vi "Msg.vi"(7 "Actor in":refnum<class "Actor.lvclass">, 11 "Actor Create Msg Strategy in":refnum<class "Actor Create Msg Strategy.lvclass">) -> (0 "error out":errorcluster, 5 "Actor out":refnum<class "Actor.lvclass">)   [LabVIEW 2021, in "Actor Create.lvlib" / "Actor Create Msg Strategy.lvclass"]
uses:
  Actor Create Msg Strategy.lvclass
  LVCAM/Actor/Actor.lvclass
  Actor Create/Actor Create.lvclass
  Actor Create Msg Strategy.lvclass/Actor Create Msg Strategy.ctl
  f99a6dc6-f889-48dc-862a-3d2cf2a0d6f5.vi
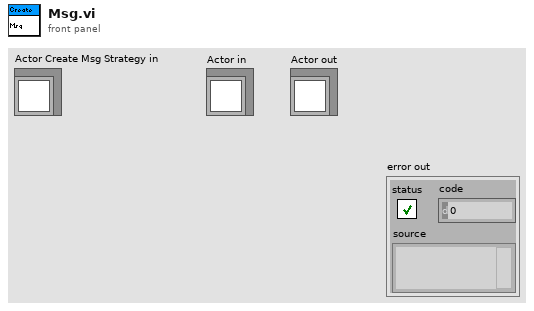
[diagram p1: front panel]
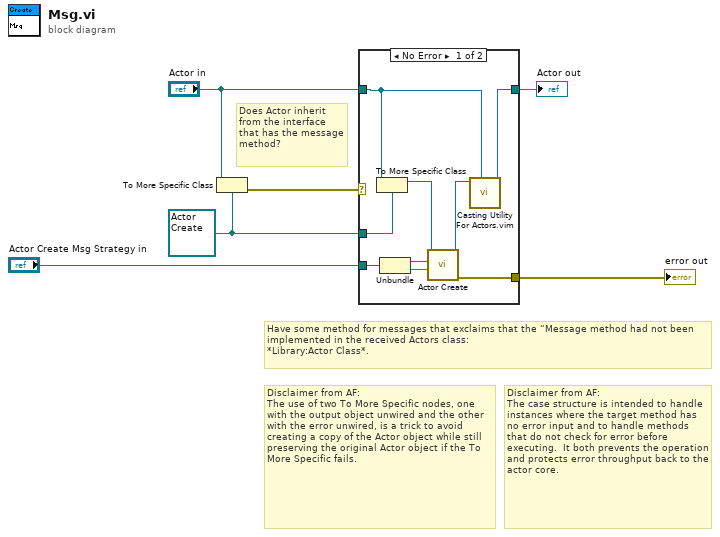
[diagram p0: block diagram]
diagram:
  w4 = refnum<class "Actor Create.lvclass"> refnum ("Create.lvlib:Create.lvclass")
  # "Does Actor inherit from the interface that has the message method?"
  # "Disclaimer from AF:\nThe use of two To More Specific nodes, one with the output object unwired and the other with the error unwired, is a trick to avoid creating a copy of the Actor object while still preserving the original Actor object if the To More Specific fails."
  # "Disclaimer from AF:\nThe case structure is intended to handle instances where the target method has no error input and to handle methods that do not check for error before executing.  It both prevents the operation and protects error throughput back to the actor core."
  # "Have some method for messages that exclaims that the “Message method had not been implemented in the received Actors class:\n*Library:Actor Class*."
  n1 = To More Specific Class(target class=w4, reference="Actor in") -> (error out=w6:errorcluster)  [unwired: 1 in, 1 out]
  n2 = case shown="No Error" w6 {
    selector: w6 -> [_ w17]
    tunnel: [w13 w17] -> w1
    tunnel: [w8 w16] -> w2
    tunnel: "Actor in" -> [w7 w16]
    tunnel: "Actor Create Msg Strategy in" -> [w12 _]
    tunnel: w4 -> [w10 _]
    frame No Error {
      n3 = To More Specific Class(target class=w10, reference=w7) -> (specific class reference=w11:refnum<class "Actor Create.lvclass">)  [unwired: 1 in, 1 out]
      n4 = Unbundle(w12) -> (w14:refnum<class "Actor.lvclass">, w15:string)
      n5 = call-dynamic "Actor Create.vi"("Nest Alias"=w15, "Nest Actor"=w14, "Actor Create in"=w11) -> ("error out"=w13:errorcluster, "Actor Create out"=w9:refnum<class "Actor Create.lvclass">)  [unwired: 7 in]
      n6 = call "Casting Utility For Actors.vim"("type"=w7, "Actor in"=w9) -> ("Actor out"=w8:refnum<class "Actor.lvclass">)  [unwired: 8 in, 1 out]
    }
    frame Error {
    }
  }
  "error out" <- w1
  "Actor out" <- w2
